vi "calibrateSignals.vi"(8 "ErrorIn":errorcluster, 11 "AccelerationDataIn":waveform(dbl)[](array[waveform])) -> (0 "ErrorOut":errorcluster, 3 "AccelerationDataOut":waveform(dbl)[](array[waveform]))   [LabVIEW 2019]
uses:
  aquireAccelerationDataVIs/Operation.ctl
  <vilib>/Analysis/baseanly.llb/Mean (DBL).vi
  <vilib>/Analysis/NI_AALBase.lvlib
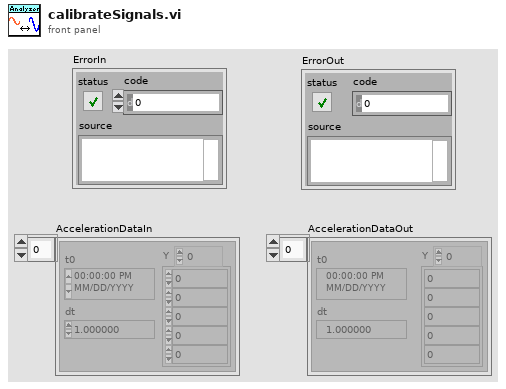
[diagram p1: front panel]
types:
  T1 = typedef "Operation.ctl" = enum16{"Initialize Connection", "Read Data", "Close Connection", "Calculate Data To m/s^2"}
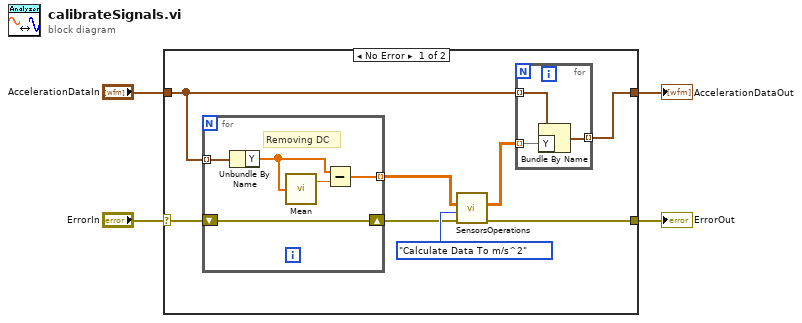
[diagram p0: block diagram]
diagram:
  n1 = case shown="No Error" "ErrorIn" {
    selector: "ErrorIn" -> [w8 w22]
    tunnel: "AccelerationDataIn" -> [w6 w21]
    tunnel: [w9 w22] -> w4
    tunnel: [w5 w21] -> w1
    frame No Error {
      n2 = for {
        tunnel: w6 -> [w19] mode=indexing
        shift-right: [w20] -> w11
        shift-left: w8 -> [w20]
        tunnel: [w16] -> w10 mode=indexing
        # "Removing DC"
        n3 = Unbundle By Name(w19) -> ("Y"=w18:dbl[])
        n4 = call-poly <vilib>:"Mean.vi"("X"=w18) -> ("mean"=w17:dbl)  [unwired: 1 out]
        n5 = Subtract(x=w18, y=w17) -> (x-y=w16:dbl[])
      }
      n6 = call "SensorsOperations.vi"("ErrorIn"=w11, "Operation"=Operation."Calculate Data To m/s^2", "RawAccelerationData In"=w10) -> ("ErrorOut"=w9:errorcluster, "Normalized Acceleration Data"=w7:dbl[][])  [unwired: 6 in, 1 out]
      n7 = for {
        tunnel: w7 -> [w14] mode=indexing
        tunnel: w6 -> [w15] mode=indexing
        tunnel: [w13] -> w5 mode=indexing
        n8 = Bundle By Name(cluster=w15, "Y"=w14) -> (w13:waveform(dbl))
      }
    }
    frame Error {
    }
  }
  "ErrorOut" <- w4
  "AccelerationDataOut" <- w1
